vi "Ordina dati npsh per report.vi"(10 "DATI NPSH":string[][](array[string]), 11 "DATI QH":string[][](array[string])) -> (3 "Array out":string[][](array[string]))   [LabVIEW 2019]
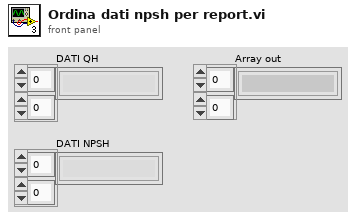
[diagram p1: front panel]
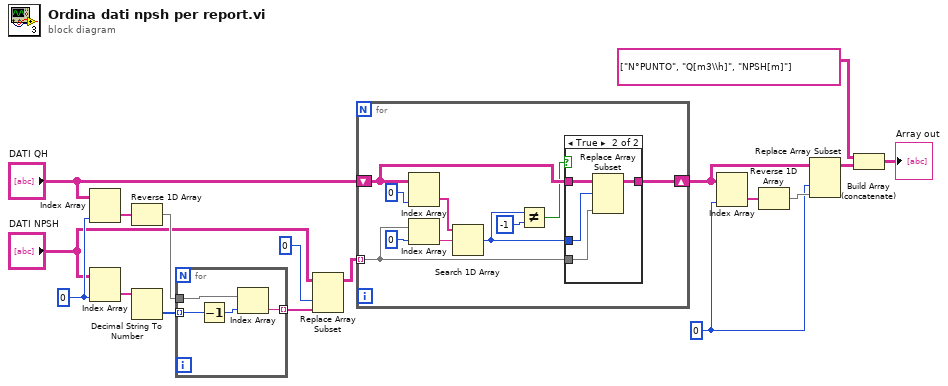
[diagram p0: block diagram]
diagram:
  w15 = 0 ("disabled index (col)")
  w5 = 0 ("disabled index (col)")
  n1 = Index Array(array="DATI QH", index (col)=w5) -> (element=w6:string[])  [unwired: 1 in]
  n2 = Index Array(array="DATI NPSH", index (col)=w5) -> (element=w8:string[])  [unwired: 1 in]
  n3 = Reverse 1D Array(array=w6) -> (reversed array=w7:string[])
  n4 = Decimal String To Number(string=w8) -> (number=w9:i32[])  [unwired: 2 in, 1 out]
  n5 = for {
    tunnel: w7 -> [w21]
    tunnel: w9 -> [w20] mode=indexing
    tunnel: [w19] -> w12 mode=indexing
    n6 = Decrement(x=w20) -> (x-1=w18:i32)
    n7 = Index Array(array=w21, index=w18) -> (element=w19:string)
  }
  n8 = Replace Array Subset(array="DATI NPSH", new element=w12, index (col)=0 ("disabled index (col)")) -> (w10:string[][])  [unwired: 1 in]
  n9 = for {
    tunnel: w10 -> [w23] mode=indexing
    shift-right: [w22] -> w14
    shift-left: "DATI QH" -> [w29]
    n10 = Index Array(array=w29, index (col)=0 ("disabled index (col)")) -> (element=w28:string[])  [unwired: 1 in]
    n11 = Index Array(array=w23, index=0) -> (element=w27:string)
    n12 = Search 1D Array(1D array=w28, element=w27) -> (index of element=w24:i32)  [unwired: 1 in]
    n13 = Not Equal?(x=w24, y=-1) -> (x != y?=w25:bool)
    n14 = case shown="True" w25 {
      tunnel: w29 -> [w32 w36]
      tunnel: w24 -> [_ w33]
      tunnel: w23 -> [_ w35]
      tunnel: [w32 w34] -> w22
      frame False {
      }
      frame True {
        n15 = Replace Array Subset(array=w36, new element=w35, index (row)=w33) -> (w34:string[][])  [unwired: 1 in]
      }
    }
  }
  n16 = Index Array(array=w14, index (col)=w15) -> (element=w13:string[])  [unwired: 1 in]
  n17 = Reverse 1D Array(array=w13) -> (reversed array=w16:string[])
  n18 = Replace Array Subset(array=w14, new element=w16, index (col)=w15) -> (w17:string[][])  [unwired: 1 in]
  n19 = Build Array (concatenate)(string[][] [["N°PUNTO", "Q[m3\\h]", "NPSH[m]"]] ("element"), w17) -> (→"Array out":string[][])
